vi "Modbus Multi-Write U32.vi"(7 "Slave Address":u8, 8 "error in (no error)":errorcluster, 9 "Input data [U32]":u32[](array[numeric]), 10 "Register Start Address":u16 format="%x", 11 "VISA resource in":refnum<visa-resource-name>) -> (0 "error out":errorcluster, 3 "VISA resource out":refnum<visa-resource-name>)   [LabVIEW 2010, in "Voegtlin_NI_SMART_Modbus_Drivers.lvlib"]
doc: "Schreibe die uebergebene Anzahl U32-Werte an die angegebene Startadresse des selektierten Geraetes.\nDer COM-Port muss dazu initialisiert sein (benutze\" Modbus Init.vi\")."
uses:
  Voegtlin_NI_SMART_Modbus_Drivers.lvlib
  Enums/Modbus Comm.ctl
panel:
  out "U16 input data to write\n(array)":u16[](array[numeric])
  # "Input Data"
  # "Internal Data"
  # "Output Data"
  # "(Inputmaske in HEX)"
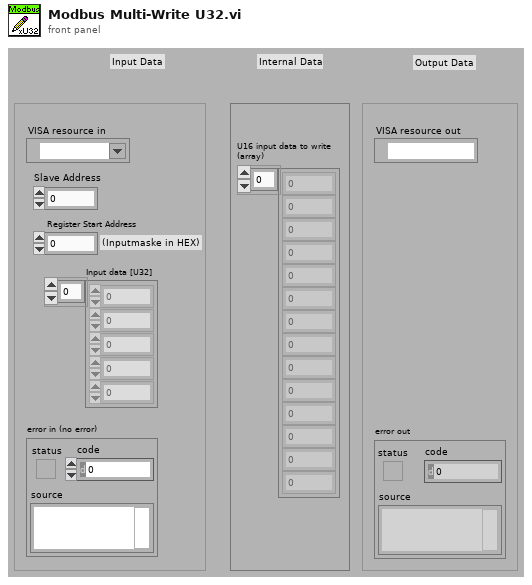
[diagram p1: front panel]
types:
  T1 = typedef "Voegtlin_NI_SMART_Modbus_Drivers.lvlib/Modbus Comm.ctl" = enum16{"Init", "Read", "Write", "Exit"}
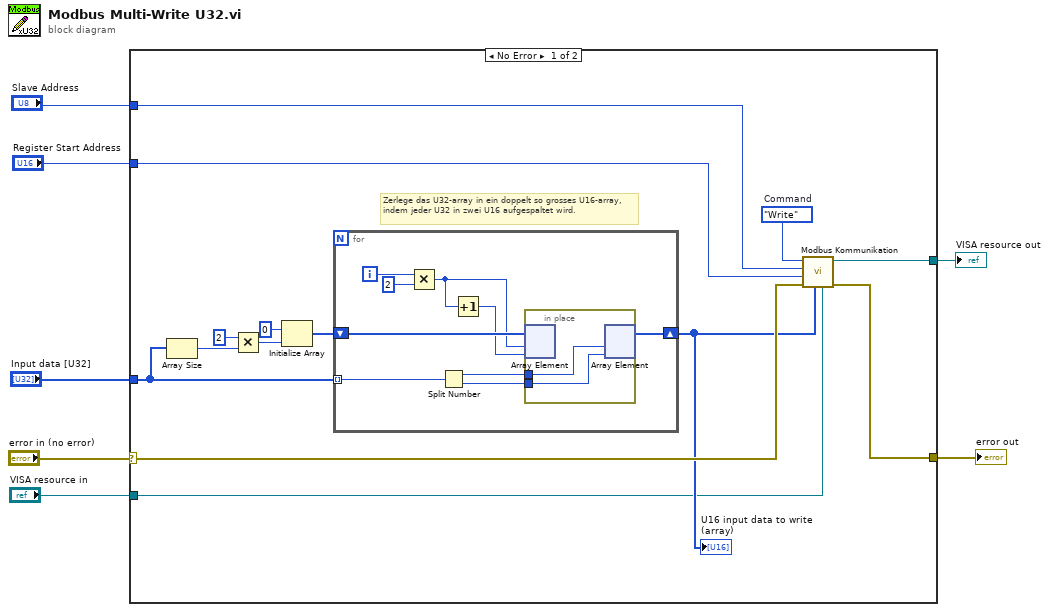
[diagram p0: block diagram]
diagram:
  n1 = case shown="No Error" "error in (no error)" {
    selector: "error in (no error)" -> [w13 w34]
    tunnel: [w20 w34] -> w7
    tunnel: "Register Start Address" -> [w11 _]
    tunnel: "Input data [U32]" -> [w14 _]
    tunnel: "Slave Address" -> [w10 _]
    tunnel: "VISA resource in" -> [w9 w33]
    tunnel: [w8 w33] -> w1
    frame No Error {
      w21 = Modbus_Comm."Write"  # Command
      # "Zerlege das U32-array in ein doppelt so grosses U16-array, indem jeder U32 in zwei U16 aufgespaltet wird."
      n2 = Array Size(array=w14) -> (size(s)=w19:i32)
      n3 = Multiply(x=2, y=w19) -> (x*y=w17:i32)
      n4 = Initialize Array(u16 0 ("x"), w17) -> (w15:u16[])
      n5 = for {
        shift-right: [w23] -> w12
        shift-left: w15 -> [w28]
        tunnel: w14 -> [w22] mode=indexing
        i -> [w30]
        n6 = Multiply(x=w30, y=2) -> (x*y=w27:i32)
        n7 = Split Number(x=w22) -> (hi(x)=w25:u16, lo(x)=w24:u16)
        n8 = Increment(x=w27) -> (x+1=w26:i32)
        n9 = in-place {
          in-place-border: w25 -> [w32]
          in-place-border: w24 -> [w31]
          n10 = in-place-array #1(w28, w27, w26) -> ()  [unwired: 2 out]
          n11 = in-place-array #1(w32, w31) -> (w23:u16[])  [unwired: 2 out]
        }
      }
      "U16 input data to write\n(array)" <- w12
      n12 = call "Modbus Kommunikation.vi"("VISA resource in"=w9, "Data In / #Reads [U16]"=w12, "error in (no error)"=w13, "Register Start Address"=w11, "Slave Address"=w10, "Command"=w21) -> ("error out"=w20:errorcluster, "VISA resource out"=w8:refnum<visa-resource-name>)  [unwired: 3 in, 1 out]
    }
    frame Error {
    }
  }
  "error out" <- w7
  "VISA resource out" <- w1
